vi "Route.vi"(8 "error in (no error)":errorcluster, 9 "Connect":bool, 10 "channel 1":string="M1H:1:5:1" caption="Route", 11 "reference in":refnum<class "Switch_Keysight_34934A.lvclass">) -> (0 "error out":errorcluster, 3 "reference in":refnum<class "Switch_Keysight_34934A.lvclass">)   [LabVIEW 2022 SP3, in "Switch_Keysight_34934A.lvlib" / "Switch_Keysight_34934A.lvclass"]
uses:
  Switch_Keysight_34934A.lvclass
  Matrix.ctl
panel:
  # "Rx:Cy:state ie R5:C2:1"
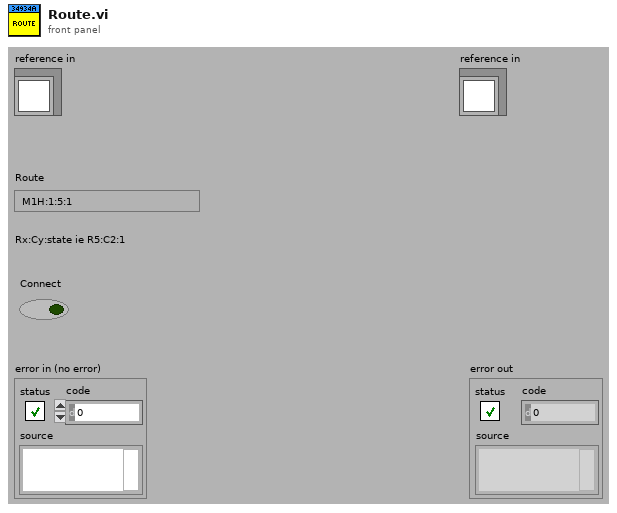
[diagram p1: front panel]
types:
  T1 = typedef "Switch_Keysight_34934A.lvlib/Switch_Keysight_34934A.lvclass/Matrix.ctl" = enum16{"M1H", "M2H", "M1L", "M2L"}
  T2 = typedef "Switch_Keysight_34934A.lvlib/Switch_Keysight_34934A.lvclass/ObjectAttributes.ctl" = cluster{"Config":T3, "VISA ref":refnum<visa-resource-name>, "M1H":bool[][], "M2H":bool[][], "M1L":bool[][], "M2L":bool[][], "route":string, "State":bool[], "StateModBit":bool[], "UpdateEvent":refnum<user-event>}
  T3 = typedef "Switch_Keysight_34934A.lvlib/Switch_Keysight_34934A.lvclass/Config.ctl" = cluster{"VISA":refnum<visa-resource-name>, "Slot":i32, "SwitchMap":cluster{"Name":string, "Route":string[], "UnRoute":string[], "Description":string, "Group":string, "IsGroup":bool}[], "Sim":bool}
  T4 = cluster{"Name":string, "Route":string[], "UnRoute":string[], "Description":string, "Group":string, "IsGroup":bool}[]
  T5 = cluster{"Name":string, "Route":string[], "UnRoute":string[], "Description":string, "Group":string, "IsGroup":bool}
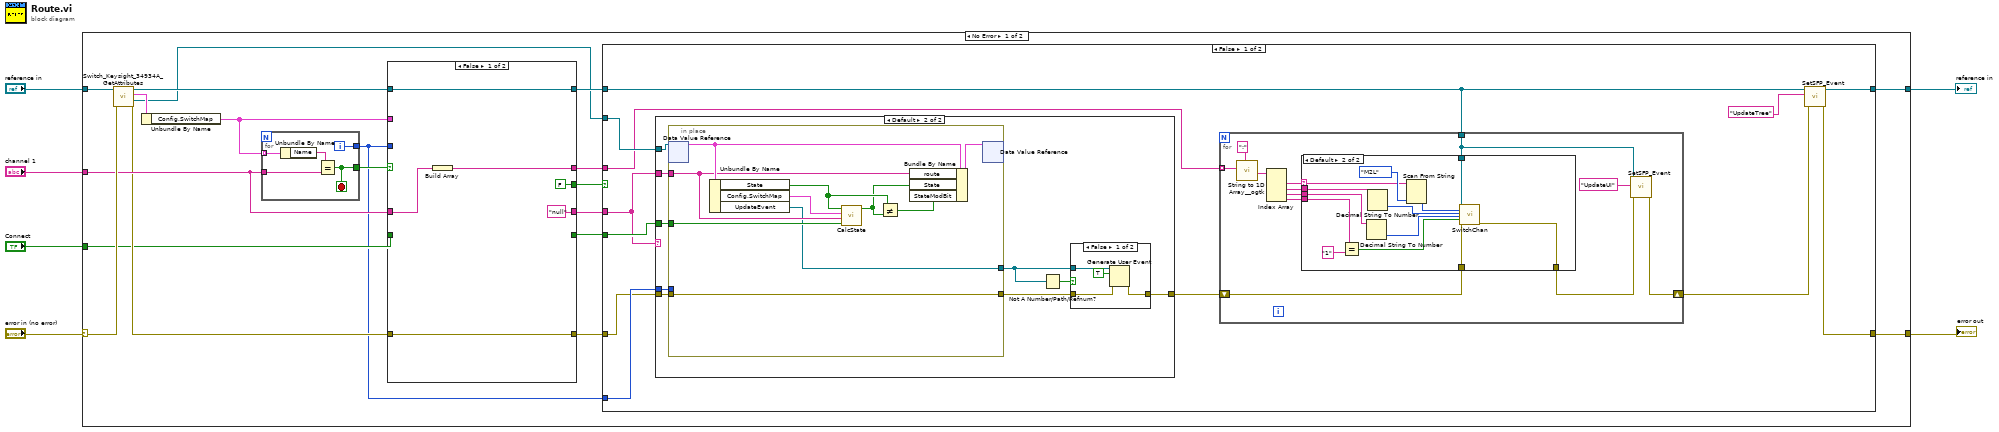
[diagram p0: block diagram]
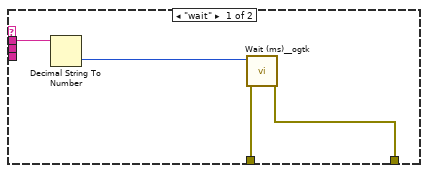
[diagram p4: hidden frame]
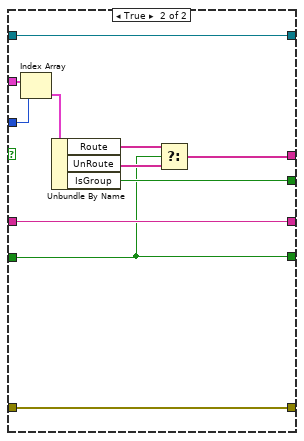
[diagram p6: hidden frame]
diagram:
  n1 = case shown="No Error" "error in (no error)" {
    selector: "error in (no error)" -> [w24 w117]
    tunnel: [w16 w117] -> w5
    tunnel: [w17 w116] -> w3
    tunnel: "reference in" -> [w25 w116]
    tunnel: "channel 1" -> [w21 _]
    tunnel: "Connect" -> [w11 _]
    frame No Error {
      n2 = call "Switch_Keysight_34934A_GetAttributes.vi"("error in (no error)"=w24, "reference in"=w25) -> ("error out"=w19:errorcluster, "DataRef"=w13:refnum<data-value>, "Data"=w23:T2, "reference out"=w18:refnum<class "Switch_Keysight_34934A.lvclass">)  [unwired: 6 in]
      n3 = Unbundle By Name(w23) -> ("Config.SwitchMap"=w20:T4)
      n4 = for {
        tunnel: w20 -> [w115] mode=indexing
        tunnel: w21 -> [w113]
        tunnel: [w112] -> w22
        tunnel: [w111] -> w7
        i -> [w111]
        stop <- w112 stop-if-true
        n5 = Unbundle By Name(w115) -> ("Name"=w114:string)
        n6 = Equal?(x=w114, y=w113) -> (x = y?=w112:bool)
      }
      n7 = case shown="False" w22 {
        tunnel: w21 -> [w97 w105]
        tunnel: w20 -> [_ w109]
        tunnel: w7 -> [_ w110]
        tunnel: w19 -> [w98 w106]
        tunnel: [w98 w106] -> w10
        tunnel: w18 -> [w99 w107]
        tunnel: [w99 w107] -> w14
        tunnel: [w96 w102] -> w15
        tunnel: ["null" ("channel 1") w105] -> w12
        tunnel: w11 -> [_ w100]
        tunnel: [FALSE ("IsGroup") w101] -> w9
        tunnel: [_ w100] -> w8
        frame False {
          n8 = Build Array(w97) -> (w96:string[])
        }
        frame True {
          n9 = Index Array(array=w109, index=w110) -> (element=w108:T5)
          n10 = Unbundle By Name(w108) -> ("Route"=w103:string[], "UnRoute"=w104:string[], "IsGroup"=w101:bool)
          n11 = Select(t=w103, s=w100, f=w104) -> (s? t:f=w102:string[])
        }
      }
      n12 = case shown="False" w9 {
        tunnel: [w31 w92] -> w17
        tunnel: [w28 w93] -> w16
        tunnel: w15 -> [w32 _]
        tunnel: w14 -> [w30 w92]
        tunnel: w13 -> [w37 _]
        tunnel: w12 -> [w26 _]
        tunnel: w10 -> [w34 w93]
        tunnel: w8 -> [w36 _]
        tunnel: w7 -> [w35 _]
        frame False {
          n13 = case shown="Default" w26 {
            tunnel: w37 -> [_ w47]
            tunnel: w36 -> [_ w46]
            tunnel: w26 -> [_ w45]
            tunnel: w35 -> [_ w44]
            tunnel: w34 -> [w38 w43]
            tunnel: [w38 w40] -> w33
            frame "null" {
            }
            frame Default {
              n14 = in-place {
                in-place-border: w43 -> [w54]
                in-place-border: [w54] -> w41
                in-place-border: w46 -> [w60]
                in-place-border: w45 -> [w59]
                in-place-border: w44 -> [_]
                in-place-border: [w53] -> w39
                n15 = in-place-dvr #1(w47) -> (w61:T2)  [unwired: 1 out]
                n16 = Unbundle By Name(w61) -> ("State"=w57:bool[], "Config.SwitchMap"=w58:T4, "UpdateEvent"=w53:refnum<user-event>)
                n17 = call "CalcState.vi"(8:"State"=w60, "Item"=w59, "Config.SwitchMap"=w58, 11:"State"=w57) -> ("State_Out"=w56:bool[])  [unwired: 7 in]
                n18 = Not Equal?(x=w57, y=w56) -> (x != y?=w55:bool[])
                n19 = Bundle By Name(cluster=w61, "route"=w59, "State"=w56, "StateModBit"=w55) -> (w62:T2)
                n20 = in-place-dvr #1(w62) -> ()  [unwired: 2 out]
              }
              n21 = Not A Number/Path/Refnum?(number/path/refnum=w39) -> (NaN/Path/Refnum?=w42:bool)
              n22 = case shown="False" w42 {
                tunnel: w41 -> [w49 w52]
                tunnel: [w50 w52] -> w40
                tunnel: w39 -> [w51 _]
                frame False {
                  n23 = Generate User Event(user event=w51, event data cluster=TRUE ("event data"), error in=w49) -> (error out=w50:errorcluster)  [unwired: 1 in, 1 out]
                }
                frame True {
                }
              }
            }
          }
          n24 = for {
            shift-right: [w64] -> w29
            shift-left: w33 -> [w74]
            tunnel: w32 -> [w73] mode=indexing
            tunnel: w30 -> [w63]
            n25 = call <userlib>:"String to 1D Array__ogtk.vi"("delimiter (Tab)"=":", "string"=w73) -> ("Array of Strings"=w71:string[])  [unwired: 9 in]
            n26 = Index Array(array=w71) -> (element #1=w67:string, element #2=w69:string, element #3=w68:string, element #4=w70:string)  [unwired: 4 in]
            n27 = case shown="Default" w67 {
              selector: w67 -> [_ w80]
              tunnel: w74 -> [w77 w91]
              tunnel: [w76 w79] -> w65
              tunnel: w63 -> [_ w89]
              tunnel: w70 -> [_ w87]
              tunnel: w69 -> [w78 w84]
              tunnel: w68 -> [_ w82]
              frame "wait" {
                n28 = Decimal String To Number(string=w78) -> (number=w75:i32)  [unwired: 2 in, 1 out]
                n29 = call <userlib>:"Wait (ms)__ogtk.vi"("error in (no error)"=w77, "milliseconds to wait"=w75) -> ("error out"=w76:errorcluster)  [unwired: 8 in, 1 out]
              }
              frame Default {
                n30 = Equal?(x=w87, y="1") -> (x = y?=w88:bool)
                n31 = Decimal String To Number(string=w82) -> (number=w81:i32)  [unwired: 2 in, 1 out]
                n32 = Decimal String To Number(string=w84) -> (number=w83:i32)  [unwired: 2 in, 1 out]
                n33 = Scan From String(input string=w80, default 1=Matrix."M2L" ("Matrix")) -> (output 1=w85:T1)  [unwired: 3 in, 3 out]
                n34 = call-dynamic "SwitchChan.vi"("reference in"=w89, "Matrix"=w85, "Row"=w83, "Column"=w81, "State"=w88, "error in (no error)"=w91) -> ("error out"=w79:errorcluster)  [unwired: 12 in, 1 out]
              }
            }
            n35 = call-dynamic "SetSFP_Event.vi"("error in (no error)"=w65, "msg"="UpdateUI", "reference in"=w63) -> ("error out"=w64:errorcluster)  [unwired: 7 in, 1 out]
          }
          n36 = call-dynamic "SetSFP_Event.vi"("error in (no error)"=w29, "msg"="UpdateTree", "reference in"=w30) -> ("error out"=w28:errorcluster, "reference out"=w31:refnum<class "Switch_Keysight_34934A.lvclass">)  [unwired: 7 in]
        }
        frame True {
        }
      }
    }
    frame Error {
    }
  }
  "error out" <- w5
  "reference in" <- w3
